vi "Read Timestamp.vi"(8 "error in (no error)":errorcluster, 11 "Sample in":refnum<class "Sample.lvclass">) -> (0 "error out":errorcluster, 2 "Timestamp Unix":u64, 3 "Sample out":refnum<class "Sample.lvclass">)   [LabVIEW 2020, in "Metrics.lvlib" / "Sample.lvclass"]
uses:
  Sample.lvclass
  Sample.lvclass/Sample.ctl
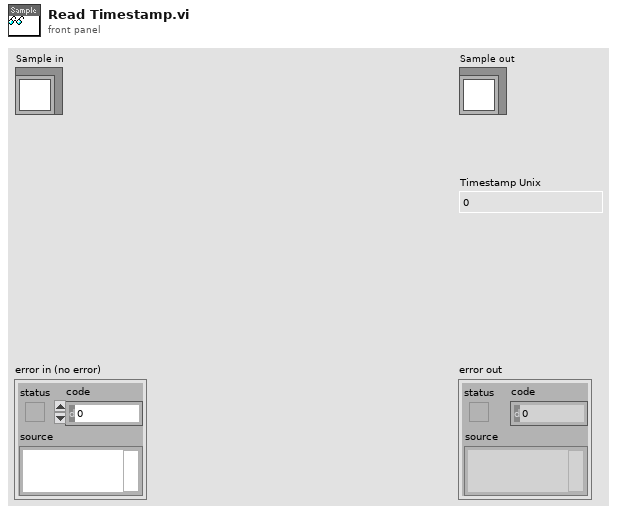
[diagram p1: front panel]
types:
  T1 = enum16{"seconds", "milliseconds", "microseconds"}
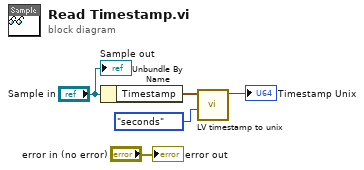
[diagram p0: block diagram]
diagram:
  n1 = Unbundle By Name("Sample in") -> ("Timestamp"=w3:timestamp)
  n2 = call "LV timestamp to unix.vi"("Precision (ms)"=T1."seconds", "Timestamp"=w3) -> ("Unix epoch time"=→"Timestamp Unix":u64)  [unwired: 9 in]
  "error out" <- "error in (no error)"
  "Sample out" <- "Sample in"
